vi "normalize_vector_cluster.vi"(1 "vector":cluster{"X":dbl, "Y":dbl}) -> (0 "normalized vector":cluster{"X":dbl, "Y":dbl})   [LabVIEW 2019]
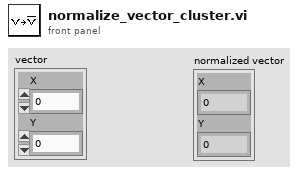
[diagram p1: front panel]
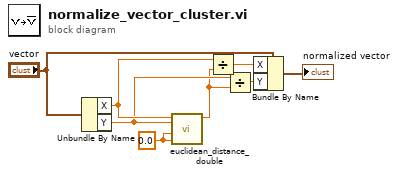
[diagram p0: block diagram]
diagram:
  w8 = 0.0
  n1 = Unbundle By Name("vector") -> ("X"=w4:dbl, "Y"=w2:dbl)
  n2 = call "euclidean_distance_double.vi"("Point 2 Y"=w8, "Point 2 X"=w8, "Point 1 Y"=w2, "Point 1 X"=w4) -> ("Distance"=w1:dbl)  [unwired: 7 in]
  n3 = Divide(x=w4, y=w1) -> (x/y=w5:dbl)
  n4 = Divide(x=w2, y=w1) -> (x/y=w3:dbl)
  n5 = Bundle By Name(cluster="vector", "X"=w5, "Y"=w3) -> (→"normalized vector":cluster{"X":dbl, "Y":dbl})
